vi "Data Types.vi"() -> ()   [LabVIEW 2021]
panel:
  out "Floating Point 2":dbl
  out "String 2":string
  out "Numeric":dbl
  in  "String":string
  out "Boolean 3":bool
  in  "Boolean":bool
  in  "Floating Point":dbl format="%#_6f"
  in  "Integer":dbl
  # "Integer does'nt exist"
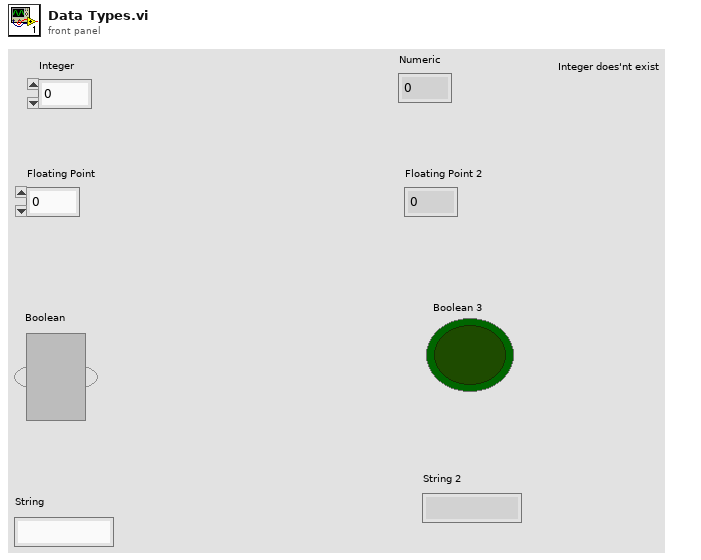
[diagram p1: front panel]
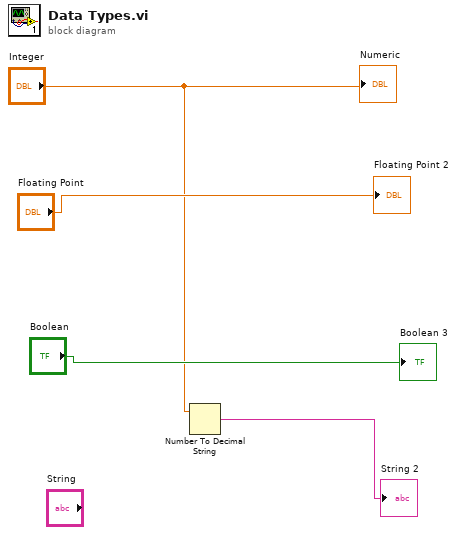
[diagram p0: block diagram]
diagram:
  n1 = Number To Decimal String(number="Integer") -> (decimal integer string=→"String 2":string)  [unwired: 1 in]
  "Boolean 3" <- "Boolean"
  "Numeric" <- "Integer"
  "Floating Point 2" <- "Floating Point"
